vi "Find Node Attribute.vi"(8 "error in":errorcluster, 10 "XPath":T1, 11 "Node":refnum<k20>) -> (0 "error out":errorcluster, 3 "Attribute":string[](array[string]))   [LabVIEW 2020, in "VI Properties Editor.lvlib"]
uses:
  VI Properties Editor.lvlib
  <vilib>/xml/NI_XML.lvlib
  <resource>/objmgr/DOMUserDefRef.rc
  <vilib>/xml/Close Reference(Node).vi
  CTLs/XPath Get Attribute.ctl
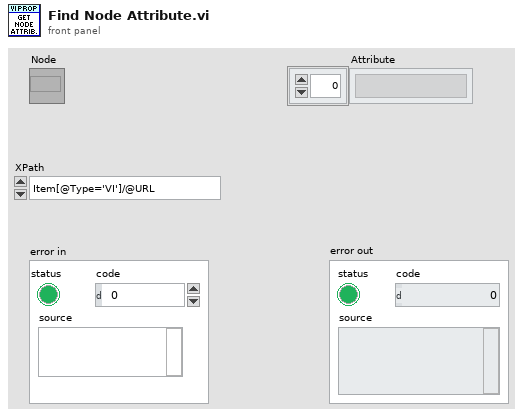
[diagram p1: front panel]
types:
  T1 = typedef "VI Properties Editor.lvlib/XPath Get Attribute.ctl" = enum16{"Item[@Type='VI']/@URL", "Item[@Type='LVClass']/@URL", "Item[@Type='Library']/@URL", "@Name"}
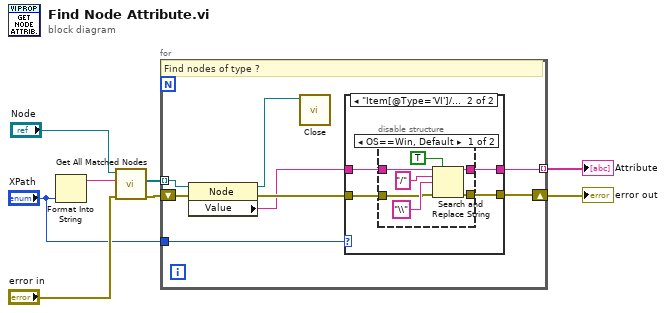
[diagram p0: block diagram]
diagram:
  n1 = Format Into String("XPath") -> (resulting string=w5:string)  [unwired: 3 in, 1 out]
  n2 = call <vilib>:"Get All Matched Nodes.vi"("error in (no error)"="error in", "XPath expression"=w5, "node in"="Node") -> ("error out"=w7:errorcluster, "node result array"=w8:refnum<k20>[])  [unwired: 6 in, 1 out]
  n3 = for {
    tunnel: w8 -> [w15] mode=indexing
    tunnel: [w14] -> w6 mode=indexing
    shift-right: [w13] -> w2
    shift-left: w7 -> [w16]
    tunnel: "XPath" -> [w9]
    # "Find nodes of type ?"
    n4 = property class="Node"(reference=w15, error in=w16) -> (reference out=w10:refnum<k20>, error out=w12:errorcluster, "Value"=w11:string)
    n5 = call-poly <vilib>:"Close.vi"("node"=w10) -> ()  [unwired: 8 in, 1 out]
    n6 = case shown="\"Item[@Type='VI']/@URL\"..\"Item[@Type='Library']/@URL\"" w9 {
      tunnel: [w17 w22] -> w14
      tunnel: [w18 w21] -> w13
      tunnel: w12 -> [w18 w20]
      tunnel: w11 -> [w17 w19]
      frame "@Name", Default {
      }
      frame "Item[@Type='VI']/@URL".."Item[@Type='Library']/@URL" {
        n7 = disable-structure shown="OS==Win, Default" {
          disable-tunnel: [w29 w31] -> w22
          disable-tunnel: w19 -> [w28 w31]
          disable-tunnel: w20 -> [w24 w30]
          disable-tunnel: [w23 w30] -> w21
          frame condition #0 (active) {
            n8 = Search and Replace String(replace all?=TRUE ("replace all? (F)"), input string=w28, search string="/", replace string="\\" ("replace string (\"\")"), error in=w24) -> (result string=w29:string, error out=w23:errorcluster)  [unwired: 3 in, 2 out]
          }
          frame condition #1 {
          }
        }
      }
    }
  }
  "Attribute" <- w6
  "error out" <- w2
